vi "Temperature_Limit.vi"() -> ()   [LabVIEW 2020]
uses:
  <vilib>/DAQmx/read.llb/DAQmx Read (Analog DBL 1Chan 1Samp).vi
  <vilib>/DAQmx/create/channels.llb/DAQmx Create Channel (AI-Voltage-Basic).vi
  <vilib>/DAQmx/configure/timing.llb/DAQmx Timing (Sample Clock).vi
  <vilib>/DAQmx/miscellaneous.llb/DAQmx Fill In Error Info.vi
panel:
  out "Waveform Chart":dbl(graph)
  out "LIMIT":bool
  in  "stop":bool
  out "error out":errorcluster
  in  "minimum value":dbl=-5.0 format="%0.2f"
  in  "maximum value":dbl=5.0 format="%0.2f"
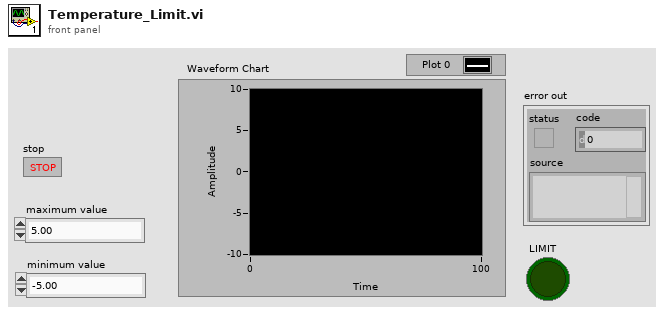
[diagram p1: front panel]
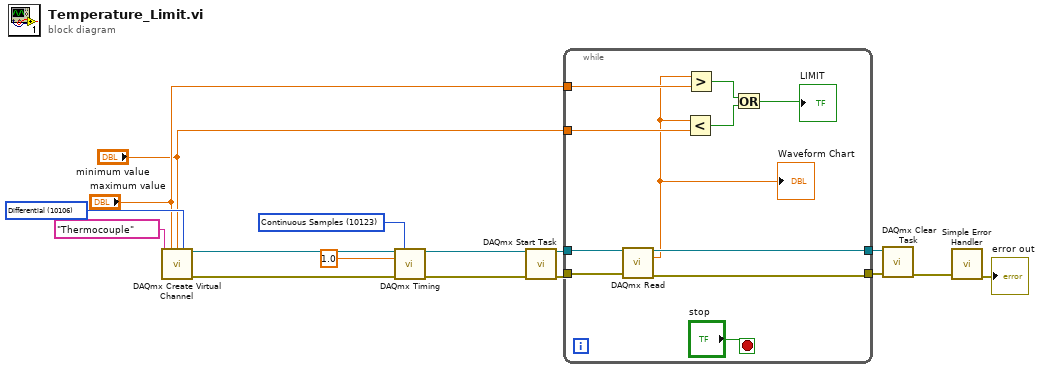
[diagram p0: block diagram]
diagram:
  w9 = 10106 items=["Default"=-1, "RSE"=10083, "NRSE"=10078, "Differential"=10106, "Pseudodifferential"=12529] ("input terminal configuration")
  w12 = 10123 items=["Finite Samples"=10178, "Continuous Samples"=10123, "Hardware Timed Single Point"=12522] ("sample mode")
  n1 = call-poly <vilib>:"DAQmx Create Virtual Channel.vi"("maximum value"="maximum value", "minimum value"="minimum value", "input terminal configuration"=w9, "physical channels"=tag "Thermocouple") -> ("task out"=w15:refnum<k21>, "error out"=w14:errorcluster)  [unwired: 10 in]
  n2 = call-poly <vilib>:"DAQmx Timing.vi"("task/channels in"=w15, "sample mode"=w12, "rate"=1.0, "error in"=w14) -> ("task out"=w10:refnum<k21>, "error out"=w11:errorcluster)  [unwired: 10 in]
  n3 = call <vilib>:"DAQmx Start Task.vi"("task/channels in"=w10, "error in"=w11) -> ("task out"=w8:refnum<k21>, "error out"=w3:errorcluster)  [unwired: 12 in]
  n4 = while {
    tunnel: w8 -> [w27]
    tunnel: [w26] -> w7
    tunnel: w3 -> [w24]
    tunnel: [w25] -> w4
    tunnel: "maximum value" -> [w22]
    tunnel: "minimum value" -> [w21]
    stop <- "stop" stop-if-true
    n5 = call-poly <vilib>:"DAQmx Read.vi"("task/channels in"=w27, "error in"=w24) -> ("task out"=w26:refnum<k21>, "data"=w17:dbl, "error out"=w25:errorcluster)  [unwired: 11 in]
    "Waveform Chart" <- w17
    n6 = Less?(x=w17, y=w21) -> (x < y?=w19:bool)
    n7 = Greater?(x=w17, y=w22) -> (0:w20:bool)
    n8 = Or(x=w20, y=w19) -> (x .or. y?=→"LIMIT":bool)
  }
  n9 = call <vilib>:"DAQmx Clear Task.vi"("task in"=w7, "error in"=w4) -> ("error out"=w6:errorcluster)  [unwired: 13 in]
  n10 = call <vilib>:"Simple Error Handler.vi"("error in (no error)"=w6) -> ("error out"=→"error out":errorcluster)  [unwired: 4 in, 4 out]
